vi "WinMan Example.vi"() -> ()   [LabVIEW 2020]
doc: "Cet exemple montre comment utiliser les VI de Window Management\n pour modifier la visu d'un UIA"
uses:
  <vilib>/Utility/miscctls.llb/LVRectTypeDef.ctl
  UI_Actor/UI_Actor Messages/UI_ShowIn_Subpanel Msg/UI_ShowIn_Subpanel Msg.lvclass/UI_ShowIn_Subpanel Msg.ctl
  UI_Actor/UI_Actor Messages/UI_ShowIn_FreeWindow Msg/UI_ShowIn_FreeWindow Msg.lvclass/UI_ShowIn_FreeWindow Msg.ctl
  support/Actor Framework.lvlibp/1abvi3w/vi.lib/ActorFramework/Message Enqueuer/Enqueue.vi
  UI_Actor/UI_Actor Messages/UI_ShowIn_Subpanel Msg/UI_ShowIn_Subpanel Msg.lvclass
  UI_Actor/UI_Actor Messages/UI_Hide Msg/UI_Hide Msg.lvclass
  UI_Actor/UI_Actor Messages/UI_ShowIn_FreeWindow Msg/UI_ShowIn_FreeWindow Msg.lvclass
  UI_Actor/UI_Actor Messages/UI_Resize Msg/UI_Resize Msg.lvclass
  UI_Actor/UI_Actor/UI_Actor.lvclass
  support/Actor Framework.lvlibp/1abvi3w/vi.lib/ActorFramework/Stop Msg/Stop Msg.lvclass
  UIA_ChildTest/UIA_ChildTest/UIA_ChildTest.lvclass
  D:/Elie/Documents/ui-actor/UI_Actor/UI_Actor/UI_Actor.lvclass
  D:/Elie/Documents/ui-actor/support/Actor Framework.lvlibp/1abvi3w/vi.lib/ActorFramework/Actor/Actor.lvclass
  D:/Elie/Documents/ui-actor/getting started/UIA_ChildTest/UIA_ChildTest/UIA_ChildTest.lvclass
panel:
  in  "Standard/Max (T=Max)":bool
  in  "Panel Bounds (if Std)":T1={"Left"=0, "Top"=0, "Right"=800, "Bottom"=600}
  in  "ShowIn SP":bool
  in  "Hide":bool
  in  "Show free":bool
  in  "stop":bool
  # "Cet exemple montre comment utiliser les VI de Window Management\n pour modifier la visu d'un UIA"
  # "Simple: 3 possibilités, 3 VIs et 3 msg pour caller les VI en remote\n- UIA en subpanel\n- UIA en fentre libre\n- UIA masqué"
  # "+ Un handle resize déja pret pour etre \nsurchargé si besoin.\n\nINFO UTILE:\nLe resize est a propagation auto sur tous les nested\n(ca n'est evidemment pas le cas des VI de positionnement)"
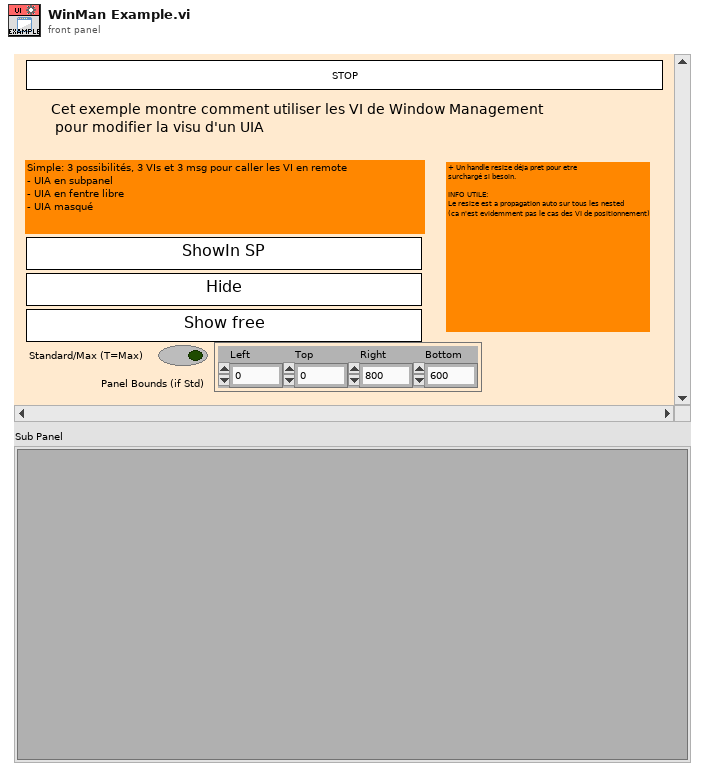
[diagram p1: front panel]
types:
  T1 = typedef "LVRectTypeDef.ctl" = cluster{"Left":i16, "Top":i16, "Right":i16, "Bottom":i16}
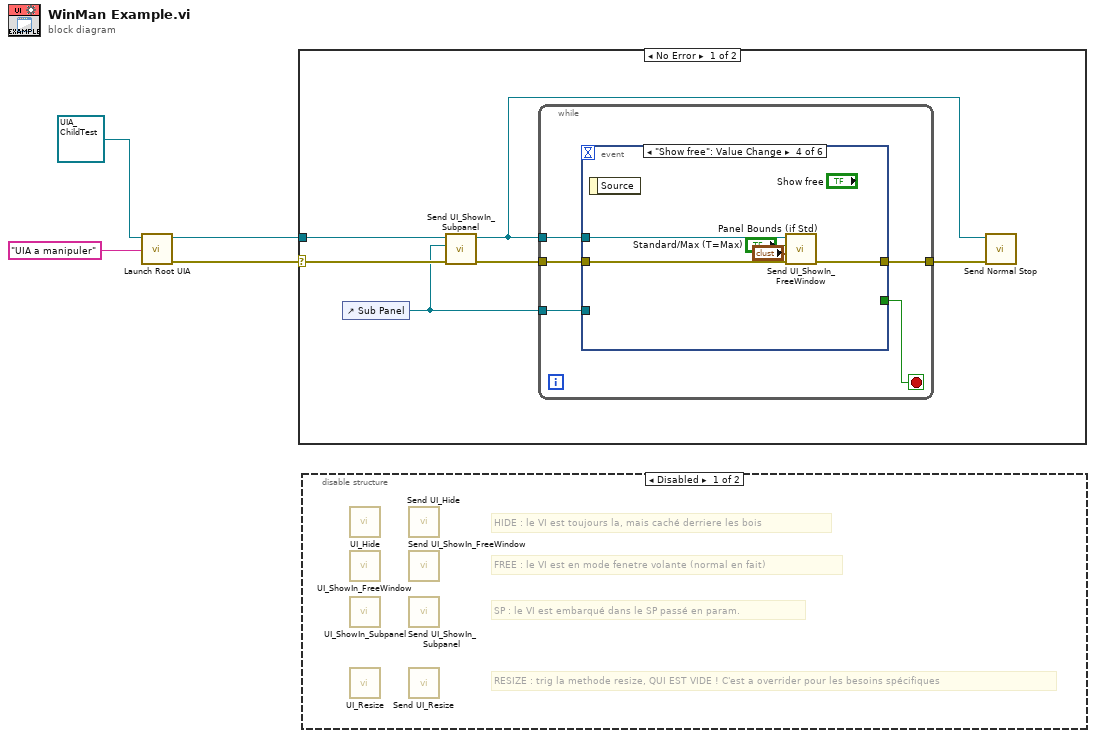
[diagram p0: block diagram]
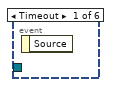
[diagram p3: hidden frame]
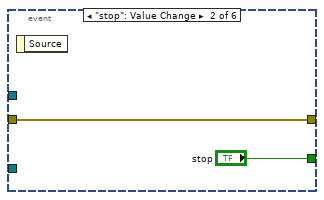
[diagram p4: hidden frame]
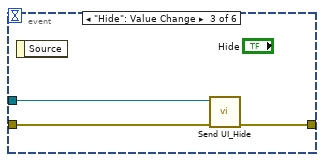
[diagram p5: hidden frame]
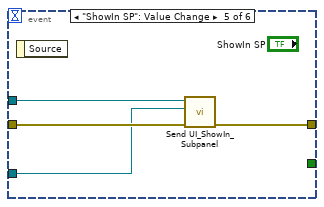
[diagram p6: hidden frame]
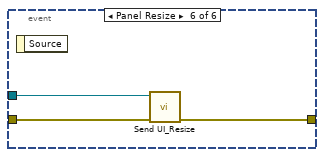
[diagram p7: hidden frame]
diagram:
  n1 = call "Launch Root UIA.vi"("Actor Name"="UIA a manipuler", "UI_Actor in"=refnum<class "UIA_ChildTest.lvclass"> refnum ("UIA_ChildTest.lvlib:UIA_ChildTest.lvclass")) -> ("error out"=w3:errorcluster, "Actor's Enqueuer"=w4:refnum<class "Message Enqueuer.lvclass">)  [unwired: 8 in]
  n2 = case shown="No Error" w3 {
    selector: w3 -> [w7 _]
    tunnel: w4 -> [w9 _]
    frame No Error {
      n3 = control-ref of="Sub Panel"() -> (w5:refnum<vi>)
      n4 = call "Send UI_ShowIn_Subpanel.vi"("error in (no error)"=w7, "Sub Panel"=w5, "Message Enqueuer"=w9) -> ("error out"=w6:errorcluster, "Message Enqueuer out"=w8:refnum<class "Message Enqueuer.lvclass">)  [unwired: 7 in]
      n5 = while {
        tunnel: w8 -> [w14]
        tunnel: [w13] -> w10
        tunnel: w6 -> [w12]
        tunnel: w5 -> [w11]
        stop <- w15 stop-if-true
        n6 = event shown="[3] \"Show free\": Value Change" {
          selector: _ -> [_ _ _ _ _ _]
          dyn-events: _ -> [_ _ _ _ _ _]
          timeout: _ -> [_ _ _ _ _ _]
          tunnel: [_ "stop" _ _ _ _] -> w15
          tunnel: w14 -> [_ _ w20 w25 w29 w32]
          tunnel: [_ w16 w18 w23 w27 w30] -> w13
          tunnel: w12 -> [_ w16 w19 w24 w28 w31]
          tunnel: w11 -> [_ _ _ _ w26 _]
          event Timeout {
            n7 = event-data() -> ()  [unwired: 1 in, 1 out]
          }
          event "stop": Value Change {
            n8 = event-data() -> ()  [unwired: 1 in, 1 out]
          }
          event "Hide": Value Change {
            n9 = event-data() -> ()  [unwired: 1 in, 1 out]
            n10 = call "Send UI_Hide.vi"("error in (no error)"=w19, "Message Enqueuer"=w20) -> ("error out"=w18:errorcluster)  [unwired: 8 in, 1 out]
          }
          event "Show free": Value Change {
            n11 = event-data() -> ()  [unwired: 1 in, 1 out]
            n12 = call "Send UI_ShowIn_FreeWindow.vi"("error in (no error)"=w24, "Panel Bounds (if Std)"="Panel Bounds (if Std)", "Standard/Max (T=Max)"="Standard/Max (T=Max)", "Message Enqueuer"=w25) -> ("error out"=w23:errorcluster)  [unwired: 6 in, 1 out]
          }
          event "ShowIn SP": Value Change {
            n13 = event-data() -> ()  [unwired: 1 in, 1 out]
            n14 = call "Send UI_ShowIn_Subpanel.vi"("error in (no error)"=w28, "Sub Panel"=w26, "Message Enqueuer"=w29) -> ("error out"=w27:errorcluster)  [unwired: 7 in, 1 out]
          }
          event Panel Resize {
            n15 = event-data() -> ()  [unwired: 1 in, 1 out]
            n16 = call "Send UI_Resize.vi"("error in (no error)"=w31, "Message Enqueuer"=w32) -> ("error out"=w30:errorcluster)  [unwired: 8 in, 1 out]
          }
        }
      }
      n17 = call "Send Normal Stop.vi"("error in (no error)"=w10, "Message Enqueuer"=w8) -> ()  [unwired: 9 in, 1 out]
    }
    frame Error {
    }
  }
  n18 = disable-structure shown="Disabled" {
    frame Disabled {
      # "RESIZE : trig la methode resize, QUI EST VIDE ! C'est a overrider pour les besoins spécifiques"
      # "SP : le VI est embarqué dans le SP passé en param."
      # "FREE : le VI est en mode fenetre volante (normal en fait)"
      # "HIDE : le VI est toujours la, mais caché derriere les bois"
      n19 = call-dynamic "UI_Hide.vi"() -> ()  [unwired: 10 in, 2 out]
      n20 = call-dynamic "UI_ShowIn_FreeWindow.vi"() -> ()  [unwired: 10 in, 2 out]
      n21 = call-dynamic "UI_ShowIn_Subpanel.vi"() -> ()  [unwired: 10 in, 2 out]
      n22 = call-dynamic "UI_Resize.vi"() -> ()  [unwired: 10 in, 2 out]
      n23 = call "Send UI_Hide.vi"() -> ()  [unwired: 10 in, 2 out]
      n24 = call "Send UI_ShowIn_FreeWindow.vi"() -> ()  [unwired: 10 in, 2 out]
      n25 = call "Send UI_ShowIn_Subpanel.vi"() -> ()  [unwired: 10 in, 2 out]
      n26 = call "Send UI_Resize.vi"() -> ()  [unwired: 10 in, 2 out]
    }
    frame Enabled {
    }
  }
